vi "Write Decimal Separator.vi"(10 "Decimal Separator":T1, 11 "StringFormatter in":refnum<class "StringFormatter.lvclass">) -> (3 "StringFormatter out":refnum<class "StringFormatter.lvclass">)   [LabVIEW 2013, in "OpenStringFormatter.lvlib" / "StringFormatter.lvclass"]
uses:
  StringFormatter.lvclass
  Localization Decimal Separator -- enum.ctl
  StringFormatter.lvclass/StringFormatter.ctl
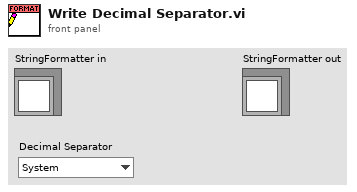
[diagram p1: front panel]
types:
  T1 = typedef "OpenStringFormatter.lvlib/StringFormatter.lvclass/Localization Decimal Separator -- enum.ctl" = enum16{"System", "Comma", "Dot"}
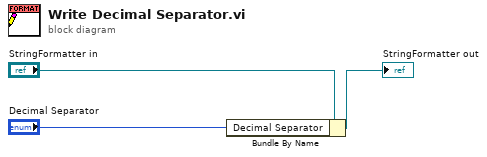
[diagram p0: block diagram]
diagram:
  n1 = Bundle By Name(cluster="StringFormatter in", "Decimal Separator"="Decimal Separator") -> (→"StringFormatter out":refnum<class "StringFormatter.lvclass">)
